vi "Actor Core.vi"(8 "error in":errorcluster, 11 "UI Actor in":refnum<class "UI Actor.lvclass">) -> (0 "error out":errorcluster, 3 "Actor out":refnum<class "Actor.lvclass">)   [LabVIEW 2024, in "UI Actor.lvlib" / "UI Actor.lvclass"]
doc: "<p>(<strong>Filename</strong>: <span class=\"dnl\">Actor Framework.lvlib:Actor.lvclass:Actor Core.vi</span>)</p>\n<p>Receives messages to the actor, reacts to them, and initiates any error handling that may shut the actor down.</p>\n<p>Descendant classes may override this VI to append parallel tasks for the actor to complete while it handles messages. Overrides use the <a href=\"nihelplauncher://docs/csh?context=lvcore_glang_udclass\">Call Parent Class Method</a> node.</p>"
uses:
  UI Actor.lvclass
  C:/Program Files/National Instruments/LabVIEW 2025/vi.lib/MGI/Panel Manager/Panel Actor/Panel Actor/Panel Actor.lvclass
  <vilib>/ActorFramework/Actor/Actor.lvclass
  Controls/Device Info.ctl
  Controls/File Info.ctl
  Controls/Device Settings.ctl
  Controls/Supported Baudrates.ctl
  Core/Object Type.ctl
  Core/Access SDO.ctl
  Core/Access PDO.ctl
  Core/Access SRDO.ctl
  D:/git/Sourcegrid-LabVIEW/dll/SourceGrid.dll
  Sourcegrid-LabVIEW/dll/SourceGrid.dll
  Controls/TX Communication Parameter.ctl
  Controls/RX Communication Parameter.ctl
  Sourcegrid-LabVIEW/source/MouseEventArgs/MouseEventArgs.lvclass
  <vilib>/MGI/Panel Manager/Panel/Panel Helper/Panel Events.ctl
  <vilib>/MGI/Panel Manager/Panel/Panel Helper/Events.ctl
  PDO Grid/PDO Grid.lvclass
  D:/git/Sourcegrid-LabVIEW/source/Grid/SourceGrid.lvclass
  <vilib>/Utility/miscctls.llb/LVRowAndColumnTypeDef.ctl
  UI Actor.lvclass/UI Actor.ctl
  Sourcegrid-LabVIEW/source/Grid/SourceGrid.lvclass/SourceGrid.ctl
  UI Actor Messages/Populate Attribute Details Msg/Populate Attribute Details Msg.lvclass/Populate Attribute Details Msg.ctl
  <vilib>/ActorFramework/Message Enqueuer/Message Enqueuer.lvclass/Message Enqueuer.ctl
  UI Actor Messages/Populate Attributes Table Msg/Populate Attributes Table Msg.lvclass/Populate Attributes Table Msg.ctl
  UI Actor Messages/Update TX Slot Display Msg/Update TX Slot Display Msg.lvclass/Update TX Slot Display Msg.ctl
  UI Actor Messages/Update RX Slot Display Msg/Update RX Slot Display Msg.lvclass/Update RX Slot Display Msg.ctl
  UI Actor Messages/Read EDS File Msg/Read EDS File Msg.lvclass/Read EDS File Msg.ctl
  <vilib>/ActorFramework/Message Enqueuer/Enqueue.vi
  UI Actor Messages/Populate Attribute Details Msg/Populate Attribute Details Msg.lvclass
  C:/Program Files/National Instruments/LabVIEW 2025/vi.lib/ActorFramework/Message/Message.lvclass
  UI Actor Messages/Populate Attributes Table Msg/Populate Attributes Table Msg.lvclass
  UI Actor Messages/Update TX Slot Display Msg/Update TX Slot Display Msg.lvclass
  UI Actor Messages/Update RX Slot Display Msg/Update RX Slot Display Msg.lvclass
  UI Actor Messages/Read EDS File Msg/Read EDS File Msg.lvclass
  <vilib>/ActorFramework/Stop Msg/Stop Msg.lvclass
  <vilib>/Utility/LVClass/Get LV Class Name.vi
  <vilib>/ActorFramework/tracing/Trace Generation/Generate Trace for Message.vi
  <vilib>/ActorFramework/Message Priority Queue/Priority Enqueue.vi
  Sourcegrid-LabVIEW/source/MouseEventArgs/Get Button.vi
  Sourcegrid-LabVIEW/source/MouseEventArgs/Get Location.vi
  <vilib>/MGI/Panel Manager/Panel Actor/Panel Actor/Panel Actor.lvclass
  UI Actor.lvlib
  Core/Electronic Datasheet.lvlib
  Sourcegrid-LabVIEW/source/Grid/SourceGrid.lvclass
  <vilib>/MGI/Panel Manager/Panel/Panel Helper/Panel Helper.lvclass
panel:
  in  "Filenames":i32(listbox)
  in  "Tab Control":T1(tab)
  out "auto":bool
  in  "Update Button":bool
  out "Concrete Node ID":string
  out "Device Settings":T2
  out "PDOs":T3
  out "File Info":T4
  out "DeviceInfo":T5
  out "Baudrates":T6
  in  "DefaultValue":string
  in  "Actual Value":string
  in  "Access SRDO":T7
  in  "Access PDO":T8
  in  "Access SDO":T9
  in  "LowLimit":string
  in  "HighLimit":string
  in  "DataType":u16(ring) items=["BOOLEAN"=1, "INTEGER8"=2, "INTEGER16"=3, "INTEGER32"=4, "UNSIGNED8"=5, "UNSIGNED16"=6, "UNSIGNED32"=7, "REAL32"=8, "VISIBLE_STRING"=9, "OCTET_STRING"=10, "UNICODE_STRING"=11, "TIME_OF_DAY"=12, "TIME_DIFFERENCE"=13, "RESERVED1"=14, "DOMAIN"=15, "INTEGER24"=16, "REAL64"=17, "INTEGER40"=18, "INTEGER48"=19, "INTEGER56"=20, "INTEGER64"=21, "UNSIGNED24"=22, "RESERVED2"=23, "UNSIGNED40"=24, "UNSIGNED48"=25, "UNSIGNED56"=26, "UNSIGNED64"=27, "RESERVED3"=28, "RESERVED4"=29, "RESERVED5"=30, "RESERVED6"=31, "PDO_COMMUNICATION_PARAMETER"=32, "PDO_MAPPING"=33, "SDO_PARAMETER"=34, "IDENTITY"=35, "RESERVED7"=36]
  out "ObjectType":T10 items=["NULL"=0, "DOMAIN"=2, "DEFTYPE"=5, "DEFSTRUCT"=6, "VAR"=7, "ARRAY"=8, "RECORD"=9]
  out "Sub-Index":string
  out "Index":string
  out "Attribute Table":string[][](table)
  out "Device Profile Specific":string[][](table)
  out "Manufacturer Specific":string[][](table)
  out "Communication Specific":string[][](table)
  in  "ParameterName":string
  in  "Description":string
  in  "Denotation":string
  in  "TX PDO Grid":refnum<k24>(container)
  out "Available Objects for TX PDO":string[][](table)
  out "TX Communication Parameter":T11 {"Type" items=["synchronous (acyclic)"=0, "synchronous (cyclic every sync)"=1, "synchronous (cyclic every 2nd SYNC)"=2, "synchronous (cyclic every 3rd SYNC)"=3, "synchronous (cyclic every 4th SYNC)"=4, "synchronous (cyclic every 240th SYNC)"=240, "reserved"=241, "reserved"=251, "RTR-only (synchronous)"=252, "RTR-only (event-driven)"=253, "event-driven (manufacturer-specific)"=254, "event-driven (device profile and application profile specific)"=255]; "COB" format="%.0x"; "Mapping" format="%.0x"; "Communication" format="%.0x"}
  in  "RX PDO Grid":refnum<k24>(container)
  out "RX Communication Parameters":T12={"Communication"=0, "Mapping"=0, "COB"=0, "Transm. Type"=254, "Inhibit"=0, "Event Timer"=0, "Sync Start"=0} {"Transm. Type" items=["synchronous"=0, "synchronous"=240, "reserved"=241, "reserved"=253, "event-driven (manufacturer-specific)"=254, "event-driven (device profile and application profile specific)"=255]; "COB" format="%.0x"; "Mapping" format="%.0x"; "Communication" format="%.0x"}
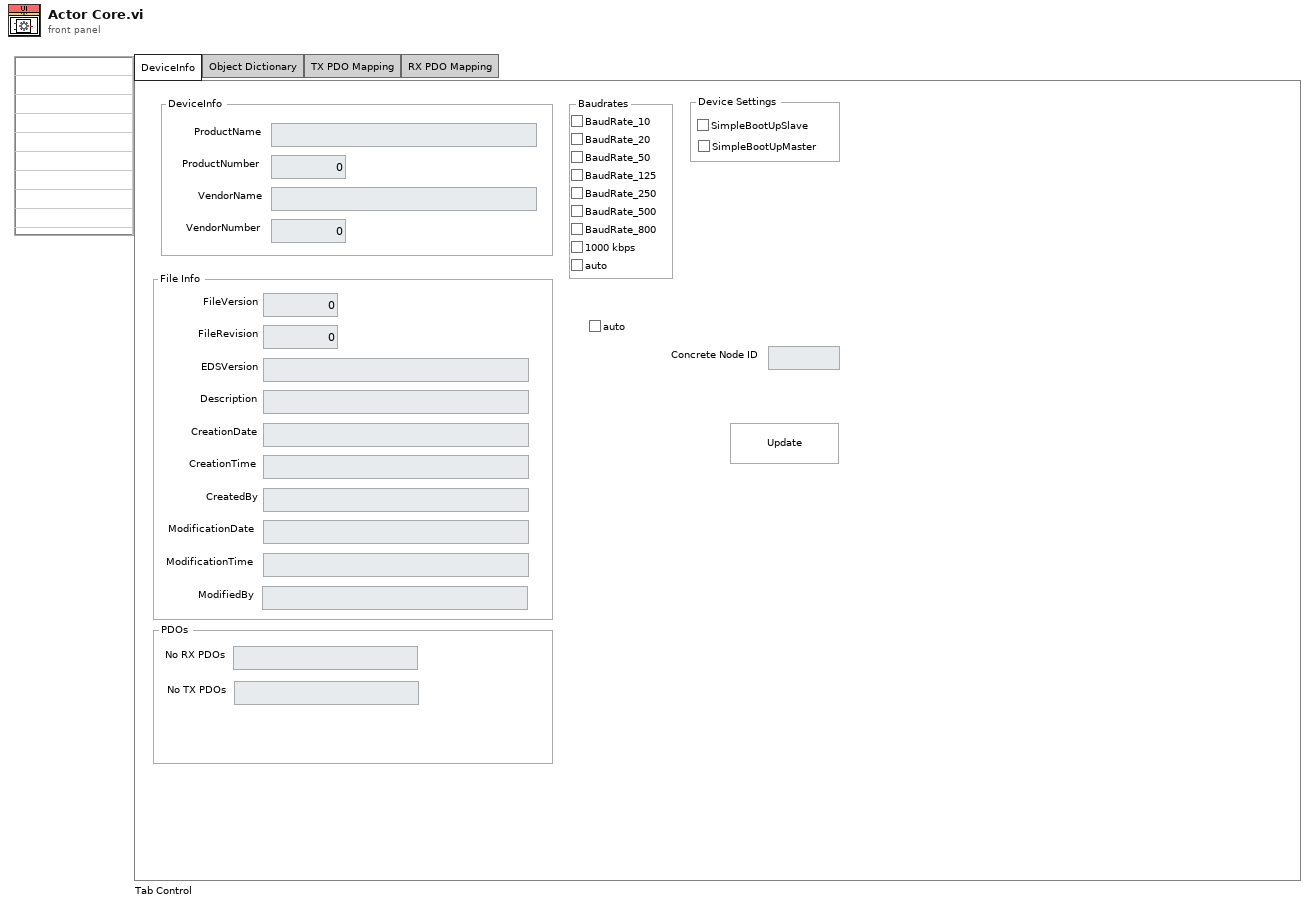
[diagram p1: front panel]
types:
  T1 = enum32{"DeviceInfo", "Object Dictionary", "TX PDO Mapping", "RX PDO Mapping"}
  T2 = typedef "UI Actor.lvlib/Device Settings.ctl" = cluster{"SimpleBootUpSlave":bool, "SimpleBootUpMaster":bool}
  T3 = cluster{"No RX PDOs":string, "No TX PDOs":string}
  T4 = typedef "UI Actor.lvlib/File Info.ctl" = cluster{"FileVersion":u8, "FileRevision":u8, "EDSVersion":string, "Description":string, "CreationDate":string, "CreationTime":string, "CreatedBy":string, "ModificationDate":string, "ModificationTime":string, "ModifiedBy":string}
  T5 = typedef "UI Actor.lvlib/Device Info.ctl" = cluster{"ProductName":string, "ProductNumber":u32, "VendorName":string, "VendorNumber":u32}
  T6 = typedef "UI Actor.lvlib/Supported Baudrates.ctl" = cluster{"BaudRate_10":bool, "BaudRate_20":bool, "BaudRate_50":bool, "BaudRate_125":bool, "BaudRate_250":bool, "BaudRate_500":bool, "BaudRate_800":bool, "BaudRate_1000":bool, "BaudRate_auto":bool}
  T7 = typedef "Electronic Datasheet.lvlib/Access SRDO.ctl" = enum16{"no", "tx", "rx", "trx"}
  T8 = typedef "Electronic Datasheet.lvlib/Access PDO.ctl" = enum16{"no", "TPDO", "RPDO", "TPDO & RPDO"}
  T9 = typedef "Electronic Datasheet.lvlib/Access SDO.ctl" = enum16{"read only", "write only", "read/write", "read/write on process input", "read/write on process output", "constant value", "no", "UNKNOWN"}
  T10 = typedef "Electronic Datasheet.lvlib/Object Type.ctl" = u8
  T11 = typedef "UI Actor.lvlib/UI Actor.lvclass/TX Communication Parameter.ctl" = cluster{"Communication":u16, "Mapping":u16, "COB":u32, "Type":u8, "Inhibit":u16, "Event Timer":u16, "Sync Start":u8}
  T12 = typedef "UI Actor.lvlib/UI Actor.lvclass/RX Communication Parameter.ctl" = cluster{"Communication":u16, "Mapping":u16, "COB":u32, "Transm. Type":u8, "Inhibit":u16, "Event Timer":u16, "Sync Start":u8}
  T13 = cluster{"Pnl Actor":refnum<event-registration>, "UI":refnum<event-registration>}
  T14 = typedef "LVRowAndColumnTypeDef.ctl" = cluster{"Row":i32, "Column":i32}
  T15 = cluster{"DeviceInfo":refnum<user-event>, "Baudrates":refnum<user-event>, "File Info":refnum<user-event>, "Device Settings":refnum<user-event>, "Filenames":refnum<user-event>, "Communication Specific":refnum<user-event>, "Manufacturer Specific":refnum<user-event>, "Device Profile Specific":refnum<user-event>, "Attribute Table":refnum<user-event>, "Attribute Details":refnum<user-event>, "TX Communication Parameter":refnum<user-event>, "RX Communication Parameter":refnum<user-event>, "Available Objects for TPDO":refnum<user-event>, "Available Objects for RPDO":refnum<user-event>}
  T16 = enum8{"Enabled", "Disabled", "Disabled and Grayed Out"}
  T17 = typedef "Rendezvous RefNum" = refnum<k1>
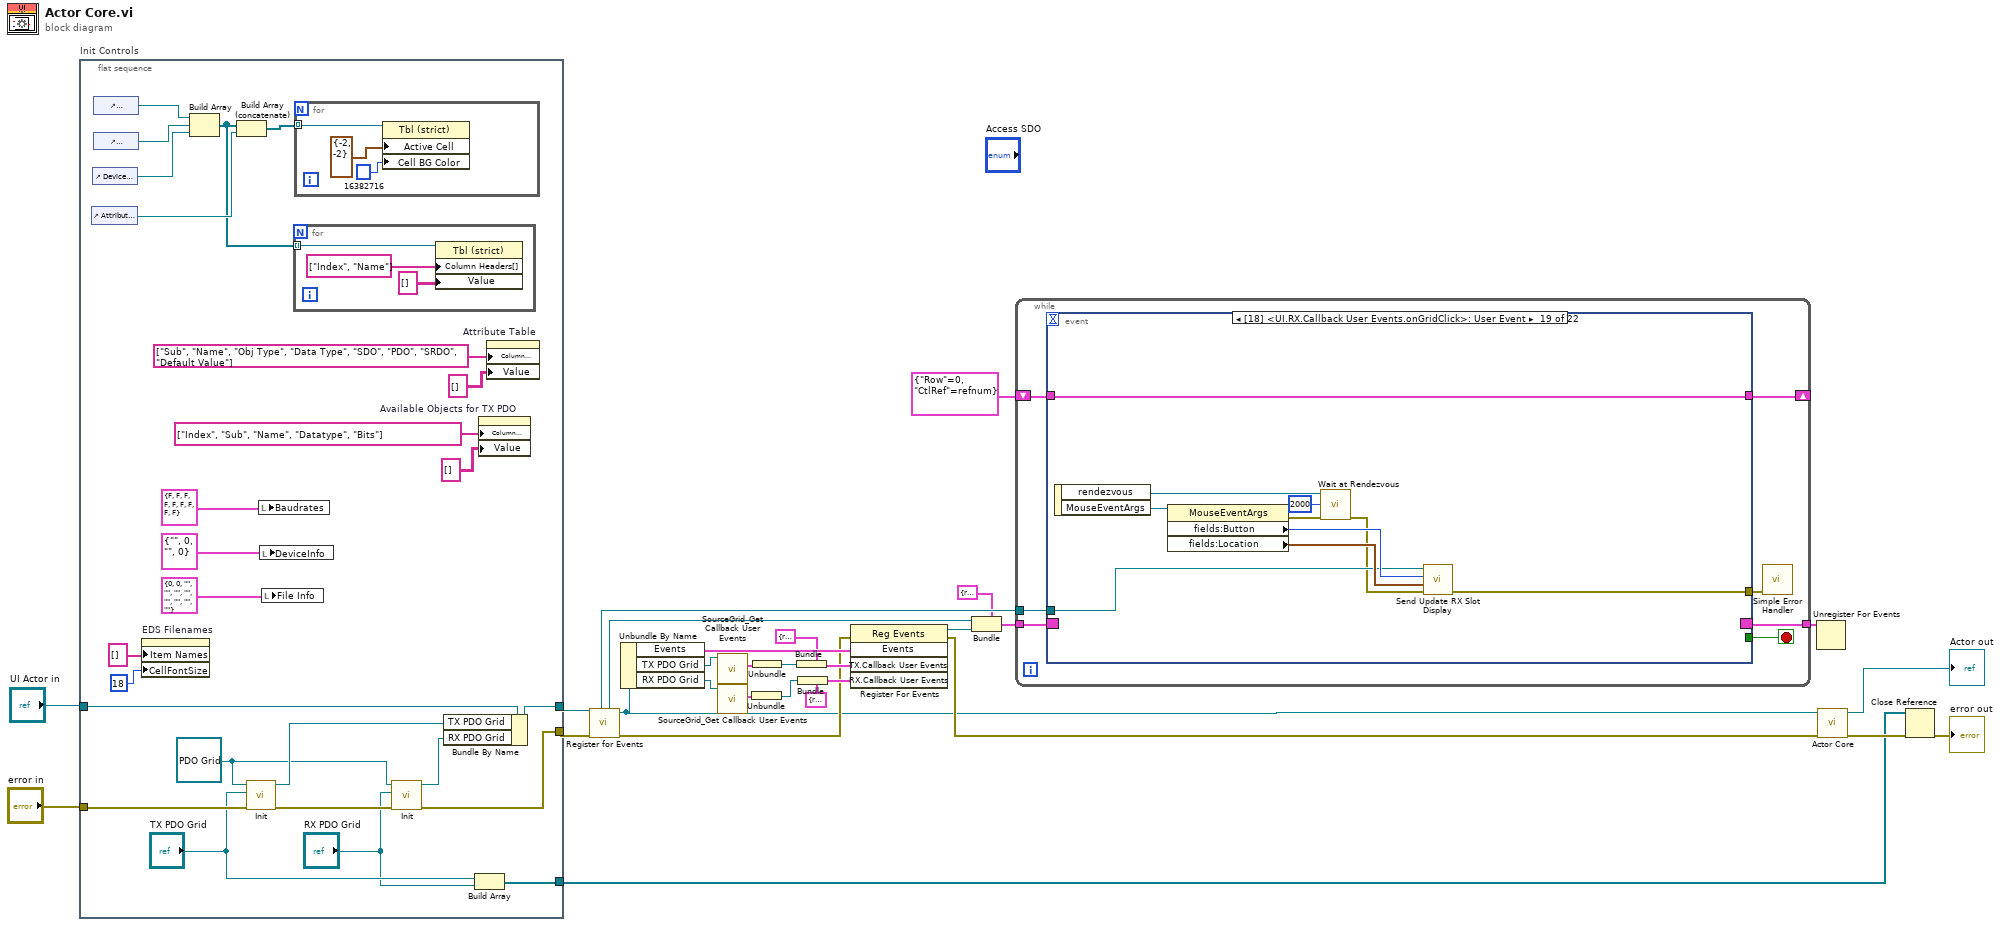
[diagram p0: block diagram]
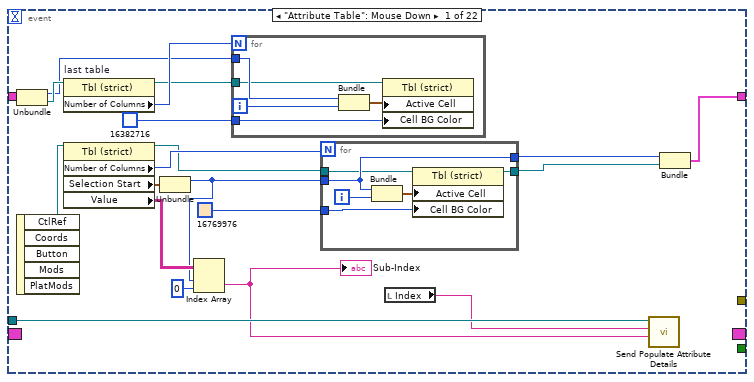
[diagram p2: hidden frame]
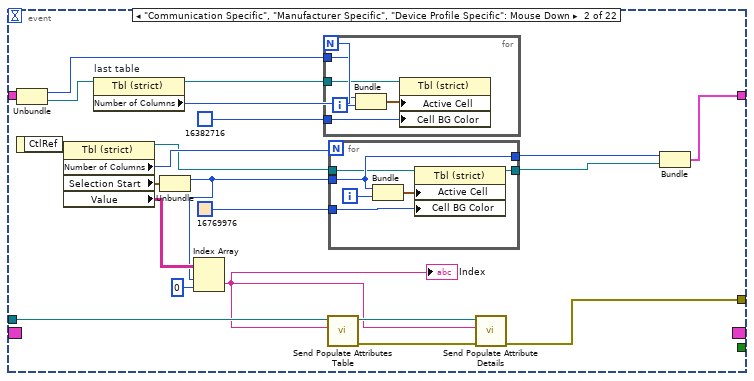
[diagram p3: hidden frame]
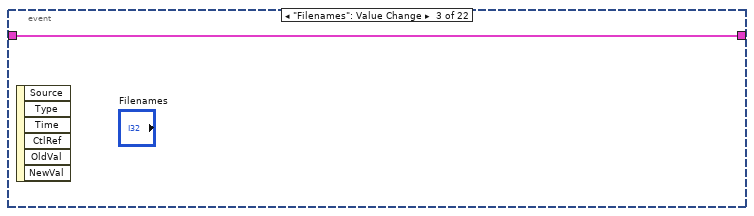
[diagram p4: hidden frame]
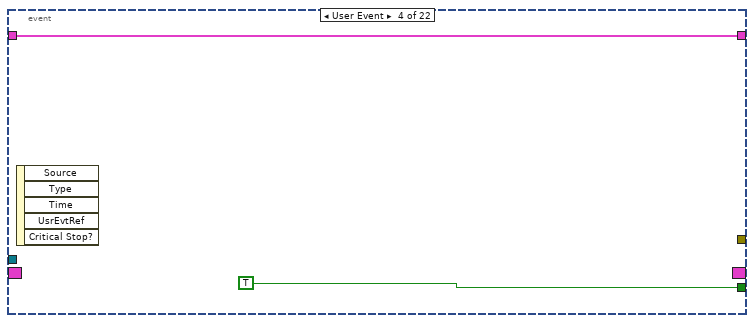
[diagram p5: hidden frame]
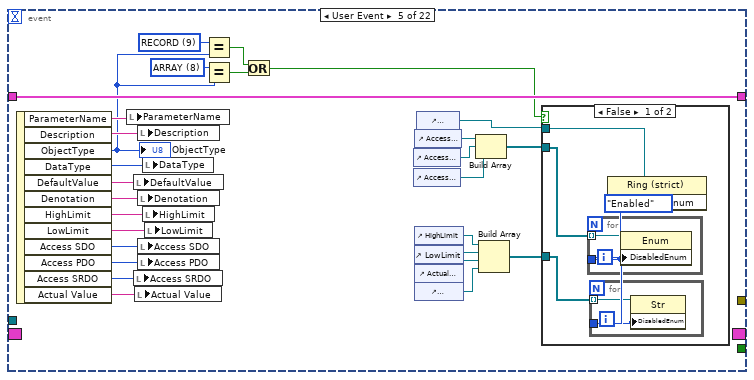
[diagram p6: hidden frame]
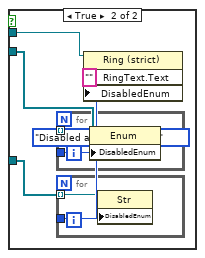
[diagram p7: hidden frame]
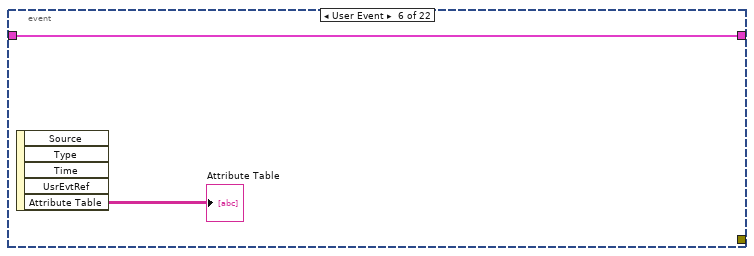
[diagram p8: hidden frame]
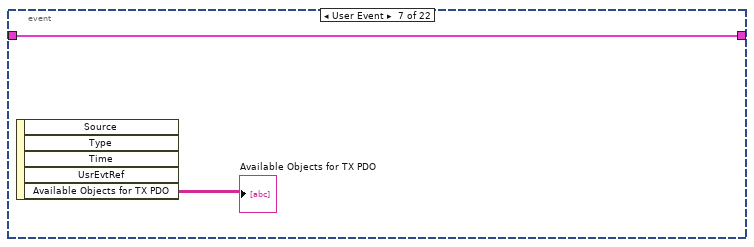
[diagram p9: hidden frame]
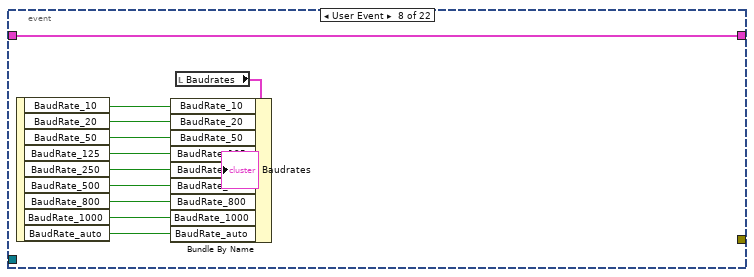
[diagram p10: hidden frame]
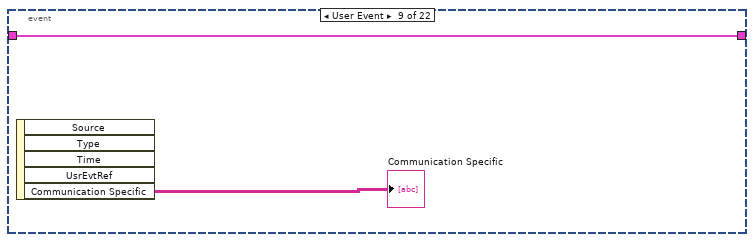
[diagram p11: hidden frame]
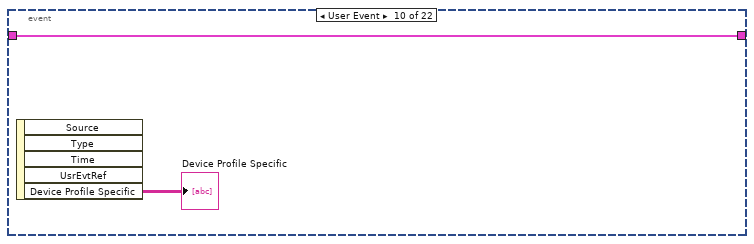
[diagram p12: hidden frame]
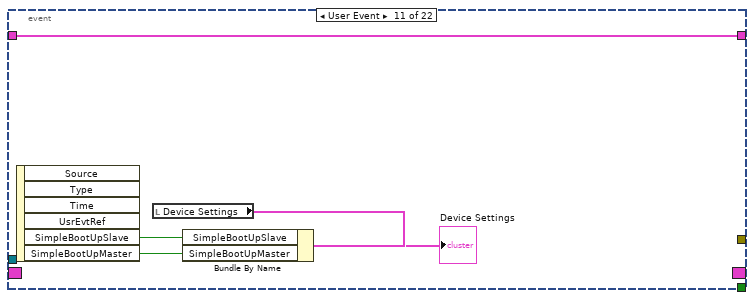
[diagram p13: hidden frame]
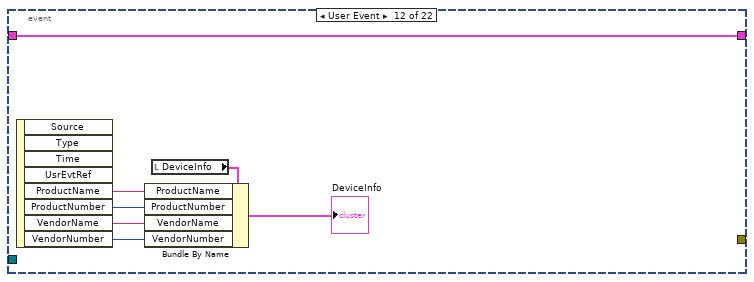
[diagram p14: hidden frame]
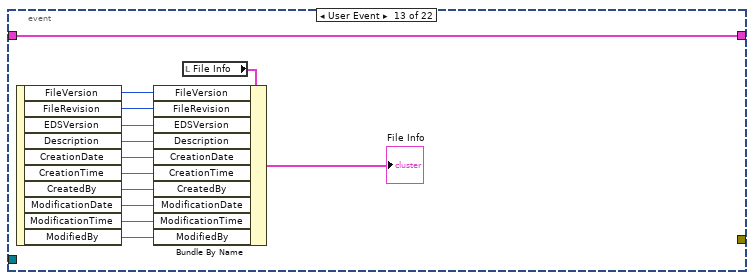
[diagram p15: hidden frame]
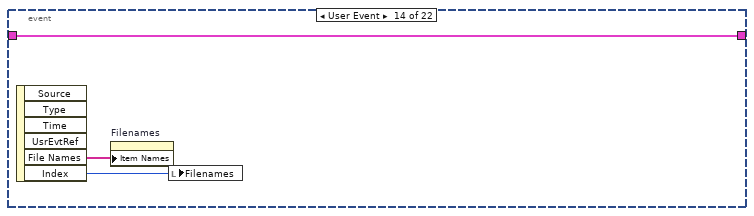
[diagram p16: hidden frame]
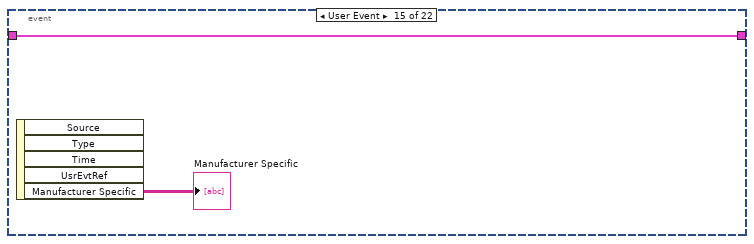
[diagram p17: hidden frame]
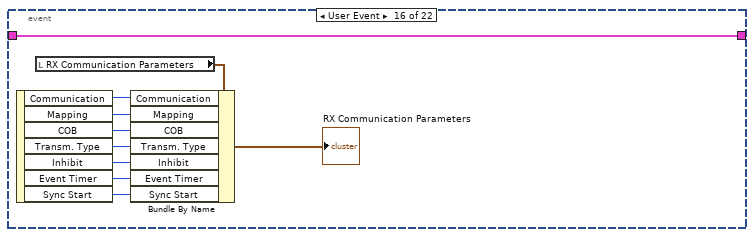
[diagram p18: hidden frame]
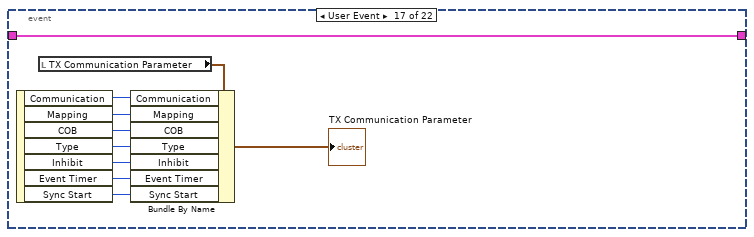
[diagram p19: hidden frame]
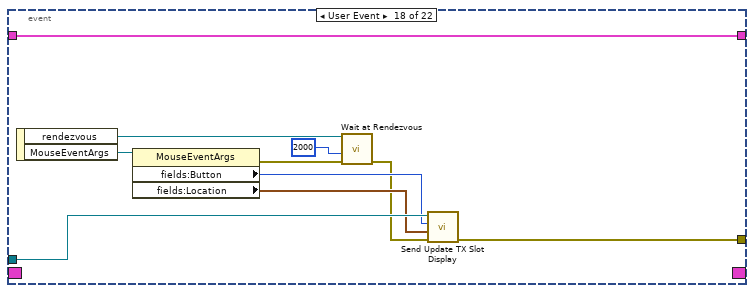
[diagram p20: hidden frame]
diagram:
  n1 = flat-sequence "Init Controls" {
    tunnel: "error in" -> [w42]
    tunnel: "UI Actor in" -> [w41]
    tunnel: [w37] -> w21
    tunnel: [w40] -> w20
    tunnel: [w30] -> w1
    frame #0 {
      w36 = refnum<class "PDO Grid.lvclass"> refnum ("PDO Grid.lvlib:PDO Grid.lvclass")
      n2 = control-ref of="Attribute Table"() -> (w44:refnum<vi>)
      n3 = control-ref of="Device Profile Specific"() -> (w46:refnum<vi>)
      n4 = control-ref of="Communication Specific"() -> (w48:refnum<vi>)
      n5 = control-ref of="Manufacturer Specific"() -> (w47:refnum<vi>)
      n6 = property on="EDS Filenames" class="LstBox (strict)"("Item Names"=string[] [], "CellFontSize"=u32 18 ("Size:Height")) -> ()  [unwired: 2 in, 2 out]
      n7 = Build Array(w48, w47, w46) -> (w43:refnum<vi>[])
      n8 = Build Array (concatenate)(w43, w44) -> (w45:refnum<vi>[])
      n9 = call-dynamic "Init.vi"("error in"=w42, "Sourcegrid Container"="TX PDO Grid", "PDO Grid in"=w36) -> ("error out"=w39:errorcluster, "PDO Grid out"=w38:refnum<class "PDO Grid.lvclass">)  [unwired: 7 in]
      n10 = local write "Baudrates"(T6 {"BaudRate_10"=FALSE, "BaudRate_20"=FALSE, "BaudRate_50"=FALSE, "BaudRate_125"=FALSE, "BaudRate_250"=FALSE, "BaudRate_500"=FALSE, "BaudRate_800"=FALSE, "BaudRate_1000"=FALSE, "BaudRate_auto"=FALSE} ("Baudrates")) -> ()
      n11 = local write "DeviceInfo"(T5 {"ProductName"="", "ProductNumber"=0, "VendorName"="", "VendorNumber"=0} ("DeviceInfo")) -> ()
      n12 = local write "File Info"(T4 {"FileVersion"=0, "FileRevision"=0, "EDSVersion"="", "Description"="", "CreationDate"="", "CreationTime"="", "CreatedBy"="", "ModificationDate"="", "ModificationTime"="", "ModifiedBy"=""} ("File Info")) -> ()
      n13 = for {
        tunnel: w43 -> [w56] mode=indexing
        n14 = property on="Property Node" class="Tbl (strict)"(reference=w56, "Column Headers[]"=string[] ["Index", "Name"] ("Compulsory Objects"), "Value"=string[][] [] ("Communication Specific")) -> ()  [unwired: 1 in, 2 out]
      }
      n15 = for {
        tunnel: w45 -> [w61] mode=indexing
        n16 = property class="Tbl (strict)"(reference=w61, "Active Cell"=T14 {"Row"=-2, "Column"=-2} ("Active Cell:Active Cell"), "Cell BG Color"=u32 16382716 ("Active Cell:Cell Background Color")) -> ()  [unwired: 1 in, 2 out]
      }
      n17 = call-dynamic "Init.vi"("error in"=w39, "Sourcegrid Container"="RX PDO Grid", "PDO Grid in"=w36) -> ("error out"=w37:errorcluster, "PDO Grid out"=w35:refnum<class "PDO Grid.lvclass">)  [unwired: 7 in]
      n18 = Bundle By Name(cluster=w41, "TX PDO Grid"=w38, "RX PDO Grid"=w35) -> (w40:refnum<class "UI Actor.lvclass">)
      n19 = Build Array("TX PDO Grid", "RX PDO Grid") -> (w30:refnum<k24>[])
      n20 = property on="Available Objects for TX PDO" class="Tbl (strict)"("Column Headers[]"=string[] ["Index", "Sub", "Name", "Datatype", "Bits"] ("Column Header Strings[]"), "Value"=string[][] [] ("Available Objects for TX PDO")) -> ()  [unwired: 2 in, 2 out]
      n21 = property on="Attribute Table" class="Tbl (strict)"("Column Headers[]"=string[] ["Sub", "Name", "Obj Type", "Data Type", "SDO", "PDO", "SRDO", "Default Value"] ("Compulsory Objects"), "Value"=string[][] [] ("Communication Specific")) -> ()  [unwired: 2 in, 2 out]
    }
  }
  n22 = call <vilib>:"Register for Events.vi"("Error In"=w21, "Panel Actor in"=w20) -> ("Error Out"=w5:errorcluster, "Panel Actor out"=w3:refnum<class "UI Actor.lvclass">, "Pnl Actor"=w27:refnum<event-registration>, "Self Enqueuer"=w26:refnum<class "Message Enqueuer.lvclass">)  [unwired: 6 in]
  n23 = Unbundle By Name(w3) -> ("Events"=w24:T15, "TX PDO Grid"=w17:refnum<class "PDO Grid.lvclass">, "RX PDO Grid"=w16:refnum<class "PDO Grid.lvclass">)
  n24 = call "SourceGrid_Get Callback User Events.vi"("SourceGrid in"=w17) -> ("Callback User Events"=w10:cluster{"onGridClick":refnum<user-event>})  [unwired: 9 in, 1 out]
  n25 = call "SourceGrid_Get Callback User Events.vi"("SourceGrid in"=w16) -> ("Callback User Events"=w15:cluster{"onGridClick":refnum<user-event>})  [unwired: 9 in, 1 out]
  n26 = Unbundle(w15) -> ("onGridClick"=w13:refnum<user-event>)
  n27 = Unbundle(w10) -> ("onGridClick"=w9:refnum<user-event>)
  n28 = Bundle(cluster=cluster{"onGridClick":refnum<user-event>} {"onGridClick"=refnum} ("TX.Callback User Events"), "onGridClick"=w9) -> (w11:cluster{"onGridClick":refnum<user-event>})
  n29 = Bundle(cluster=cluster{"onGridClick":refnum<user-event>} {"onGridClick"=refnum} ("RX.Callback User Events"), "onGridClick"=w13) -> (w14:cluster{"onGridClick":refnum<user-event>})
  n30 = register-events(error in=w5, w24, w11, w14) -> (reference out=w7:refnum<event-registration>, error out=w4:errorcluster)  [unwired: 1 in]
  n31 = Bundle(cluster=T13 {"Pnl Actor"=refnum, "UI"=refnum}, "Pnl Actor"=w27, "UI"=w7) -> (w25:T13)
  n32 = while {
    tunnel: w25 -> [w67]
    tunnel: w26 -> [w66]
    shift-right: [w65] -> _
    shift-left: cluster{"Row":i32, "CtlRef":refnum<vi>} {"Row"=0, "CtlRef"=refnum} -> [w64]
    tunnel: [w63] -> w18
    stop <- w68 stop-if-true
    n33 = event shown="[18] <UI.RX.Callback User Events.onGridClick>: User Event" {
      selector: w67 -> [_ _ _ _ _ _ _ _ _ _ _ _ _ _ _ _ _ _ _ _ _ _]
      dyn-events: [_ _ _ _ _ _ _ _ _ _ _ _ _ _ _ _ _ _ _ _ _ _] -> w63
      timeout: _ -> [_ _ _ _ _ _ _ _ _ _ _ _ _ _ _ _ _ _ _ _ _ _]
      tunnel: [_ _ _ TRUE _ _ _ _ _ _ _ _ _ _ _ _ _ _ _ _ _ _] -> w68
      tunnel: w66 -> [w73 w106 _ _ _ _ _ _ _ _ _ _ _ _ _ _ _ w258 w266 w273 w298 _]
      tunnel: [w78 w111 w133 w134 w163 w181 w183 w185 w198 w199 w201 w206 w213 w226 w229 w232 w241 w260 w264 w272 w297 w300] -> w65
      tunnel: w64 -> [w87 w120 w133 w134 w163 w181 w183 w185 w198 w199 w201 w206 w213 w226 w229 w232 w241 w260 w264 w272 w297 w300]
      tunnel: [_ w100 _ _ _ _ _ _ _ _ _ _ _ _ _ _ _ w256 w265 w271 _ _] -> w62
      event "Attribute Table": Mouse Down {
        n34 = Unbundle(w87) -> ("Row"=w79:i32, "CtlRef"=w80:refnum<vi>)
        n35 = event-data() -> ("CtlRef"=w75:refnum<vi>)  [unwired: 1 in, 4 out]
        n36 = property on="last table" class="Tbl (strict)"(reference=w80) -> (reference out=w76:refnum<vi>, "Number of Columns"=w81:u32)  [unwired: 1 in, 1 out]
        n37 = property class="Tbl (strict)"(reference=w75) -> (reference out=w83:refnum<vi>, "Number of Columns"=w86:u32, "Selection Start"=w88:T14, "Value"=w74:string[][])  [unwired: 1 in, 1 out]
        n38 = Unbundle(w88) -> ("Row"=w71:i32)  [unwired: 1 out]
        n39 = Index Array(array=w74, index (row)=w71, index (col)=0) -> (element=w69:string)
        "Sub-Index" <- w69
        n40 = for {
          N: w81 -> [_]
          tunnel: u32 16382716 ("Active Cell:Cell Background Color") -> [w99]
          tunnel: w79 -> [w96]
          tunnel: w76 -> [w95]
          i -> [w98]
          n41 = Bundle("Row"=w96, w98) -> (w97:cluster{"Row":i32, i32})  [unwired: 1 in]
          n42 = property class="Tbl (strict)"(reference=w95, "Active Cell"=w97, "Cell BG Color"=w99) -> ()  [unwired: 1 in, 2 out]
        }
        n43 = for {
          N: w86 -> [_]
          tunnel: w71 -> [w93]
          tunnel: u32 16769976 -> [w92]
          tunnel: [w93] -> w84
          tunnel: w83 -> [w90]
          tunnel: [w89] -> w77
          i -> [w94]
          n44 = Bundle("Row"=w93, w94) -> (w91:cluster{"Row":i32, i32})  [unwired: 1 in]
          n45 = property class="Tbl (strict)"(reference=w90, "Active Cell"=w91, "Cell BG Color"=w92) -> (reference out=w89:refnum<vi>)  [unwired: 1 in, 1 out]
        }
        n46 = local read "Index"() -> (w70:string)
        n47 = call "Send Populate Attribute Details.vi"("Sub-Index"=w69, "Index"=w70, "Message Enqueuer"=w73) -> ()  [unwired: 7 in, 2 out]
        n48 = Bundle("Row"=w84, "CtlRef"=w77) -> (w78:cluster{"Row":i32, "CtlRef":refnum<vi>})  [unwired: 1 in]
      }
      event "Communication Specific", "Manufacturer Specific", "Device Profile Specific": Mouse Down {
        n49 = Unbundle(w120) -> ("Row"=w112:i32, "CtlRef"=w113:refnum<vi>)
        n50 = event-data() -> ("CtlRef"=w108:refnum<vi>)  [unwired: 1 in]
        n51 = property class="Tbl (strict)"(reference=w108) -> (reference out=w116:refnum<vi>, "Number of Columns"=w119:u32, "Selection Start"=w121:T14, "Value"=w107:string[][])  [unwired: 1 in, 1 out]
        n52 = property on="last table" class="Tbl (strict)"(reference=w113) -> (reference out=w109:refnum<vi>, "Number of Columns"=w114:u32)  [unwired: 1 in, 1 out]
        n53 = Unbundle(w121) -> ("Row"=w104:i32)  [unwired: 1 out]
        n54 = Index Array(array=w107, index (row)=w104, index (col)=0) -> (element=w102:string)
        "Index" <- w102
        n55 = for {
          N: w114 -> [_]
          tunnel: u32 16382716 ("Active Cell:Cell Background Color") -> [w132]
          tunnel: w112 -> [w129]
          tunnel: w109 -> [w128]
          i -> [w131]
          n56 = Bundle("Row"=w129, w131) -> (w130:cluster{"Row":i32, i32})  [unwired: 1 in]
          n57 = property class="Tbl (strict)"(reference=w128, "Active Cell"=w130, "Cell BG Color"=w132) -> ()  [unwired: 1 in, 2 out]
        }
        n58 = call "Send Populate Attributes Table.vi"("Index"=w102, "Message Enqueuer"=w106) -> ("error out"=w101:errorcluster, "Message Enqueuer out"=w103:refnum<class "Message Enqueuer.lvclass">)  [unwired: 8 in]
        n59 = for {
          N: w119 -> [_]
          tunnel: w104 -> [w126]
          tunnel: u32 16769976 -> [w125]
          tunnel: [w126] -> w117
          tunnel: w116 -> [w123]
          tunnel: [w122] -> w110
          i -> [w127]
          n60 = Bundle("Row"=w126, w127) -> (w124:cluster{"Row":i32, i32})  [unwired: 1 in]
          n61 = property class="Tbl (strict)"(reference=w123, "Active Cell"=w124, "Cell BG Color"=w125) -> (reference out=w122:refnum<vi>)  [unwired: 1 in, 1 out]
        }
        n62 = call "Send Populate Attribute Details.vi"("error in (no error)"=w101, "Index"=w102, "Message Enqueuer"=w103) -> ("error out"=w100:errorcluster)  [unwired: 7 in, 1 out]
        n63 = Bundle("Row"=w117, "CtlRef"=w110) -> (w111:cluster{"Row":i32, "CtlRef":refnum<vi>})  [unwired: 1 in]
      }
      event "Filenames": Value Change {
        n64 = event-data() -> ()  [unwired: 1 in, 6 out]
      }
      event User Event {
        n65 = event-data() -> ()  [unwired: 1 in, 5 out]
      }
      event User Event {
        w147 = T10 9 items=["NULL"=0, "DOMAIN"=2, "DEFTYPE"=5, "DEFSTRUCT"=6, "VAR"=7, "ARRAY"=8, "RECORD"=9] ("x")
        w148 = T10 8 items=["NULL"=0, "DOMAIN"=2, "DEFTYPE"=5, "DEFSTRUCT"=6, "VAR"=7, "ARRAY"=8, "RECORD"=9] ("x")
        n66 = event-data() -> ("ParameterName"=w162:string, "Description"=w161:string, "ObjectType"=w149:T10, "DataType"=w160:u16, "DefaultValue"=w159:string, "Denotation"=w158:string, "HighLimit"=w157:string, "LowLimit"=w156:string, "Access SDO"=w155:T9, "Access PDO"=w154:T8, "Access SRDO"=w153:T7, "Actual Value"=w152:string)  [unwired: 1 in]
        "ObjectType" <- w149
        n67 = local write "ParameterName"(w162) -> ()
        n68 = local write "DefaultValue"(w159) -> ()
        n69 = local write "Access SRDO"(w153) -> ()
        n70 = local write "Actual Value"(w152) -> ()
        n71 = local write "Description"(w161) -> ()
        n72 = local write "Denotation"(w158) -> ()
        n73 = local write "Access SDO"(w155) -> ()
        n74 = local write "Access PDO"(w154) -> ()
        n75 = local write "DataType"(w160) -> ()
        n76 = local write "HighLimit"(w157) -> ()
        n77 = local write "LowLimit"(w156) -> ()
        n78 = Equal?(x=w147, y=w149) -> (x = y?=w150:bool)
        n79 = Equal?(x=w148, y=w149) -> (x = y?=w151:bool)
        n80 = Or(x=w150, y=w151) -> (x .or. y?=w137:bool)
        n81 = control-ref of="Access PDO"() -> (w145:refnum<vi>)
        n82 = control-ref of="Access SRDO"() -> (w144:refnum<vi>)
        n83 = control-ref of="Access SDO"() -> (w146:refnum<vi>)
        n84 = control-ref of="HighLimit"() -> (w139:refnum<vi>)
        n85 = control-ref of="LowLimit"() -> (w140:refnum<vi>)
        n86 = control-ref of="Actual Value"() -> (w141:refnum<vi>)
        n87 = control-ref of="DefaultValue"() -> (w142:refnum<vi>)
        n88 = control-ref of="ObjectType"() -> (w136:refnum<vi>)
        n89 = Build Array(w146, w145, w144) -> (w143:refnum<vi>[])
        n90 = Build Array(w139, w140, w141, w142) -> (w138:refnum<vi>[])
        n91 = case shown="False" w137 {
          tunnel: w143 -> [w166 w176]
          tunnel: w138 -> [w167 w175]
          tunnel: w136 -> [w165 w174]
          frame False {
            w164 = T16."Enabled" ("Disabled")
            n92 = for {
              tunnel: w166 -> [w171] mode=indexing
              tunnel: w164 -> [w170]
              n93 = property on="Property Node" class="Enum"(reference=w171, "DisabledEnum"=w170) -> ()  [unwired: 1 in, 2 out]
            }
            n94 = for {
              tunnel: w167 -> [w169] mode=indexing
              tunnel: w164 -> [w168]
              n95 = property on="Property Node" class="Str"(reference=w169, "DisabledEnum"=w168) -> ()  [unwired: 1 in, 2 out]
            }
            n96 = property on="Property Node" class="Ring (strict)"(reference=w165, "DisabledEnum"=w164) -> ()  [unwired: 1 in, 2 out]
          }
          frame True {
            w172 = T16."Disabled and Grayed Out" ("Disabled")
            n97 = for {
              tunnel: w176 -> [w180] mode=indexing
              tunnel: w172 -> [w179]
              n98 = property on="Property Node" class="Enum"(reference=w180, "DisabledEnum"=w179) -> ()  [unwired: 1 in, 2 out]
            }
            n99 = for {
              tunnel: w175 -> [w178] mode=indexing
              tunnel: w172 -> [w177]
              n100 = property on="Property Node" class="Str"(reference=w178, "DisabledEnum"=w177) -> ()  [unwired: 1 in, 2 out]
            }
            n101 = property on="Property Node" class="Ring (strict)"(reference=w174, "RingText.Text"="" ("Ring Text.Text"), "DisabledEnum"=w172) -> ()  [unwired: 1 in, 2 out]
          }
        }
      }
      event User Event {
        n102 = event-data() -> ("Attribute Table"=→"Attribute Table":string[][])  [unwired: 1 in, 4 out]
      }
      event User Event {
        n103 = event-data() -> ("Available Objects for TX PDO"=→"Available Objects for TX PDO":string[][])  [unwired: 1 in, 4 out]
      }
      event User Event {
        n104 = event-data() -> ("BaudRate_10"=w195:bool, "BaudRate_20"=w194:bool, "BaudRate_50"=w193:bool, "BaudRate_125"=w192:bool, "BaudRate_250"=w191:bool, "BaudRate_500"=w190:bool, "BaudRate_800"=w189:bool, "BaudRate_1000"=w188:bool, "BaudRate_auto"=w186:bool)  [unwired: 1 in]
        n105 = local read "Baudrates"() -> (w196:T6)
        n106 = Bundle By Name(cluster=w196, "BaudRate_10"=w195, "BaudRate_20"=w194, "BaudRate_50"=w193, "BaudRate_125"=w192, "BaudRate_250"=w191, "BaudRate_500"=w190, "BaudRate_800"=w189, "BaudRate_1000"=w188, "BaudRate_auto"=w186) -> (→"Baudrates":T6)
      }
      event User Event {
        n107 = event-data() -> ("Communication Specific"=→"Communication Specific":string[][])  [unwired: 1 in, 4 out]
      }
      event User Event {
        n108 = event-data() -> ("Device Profile Specific"=→"Device Profile Specific":string[][])  [unwired: 1 in, 4 out]
      }
      event User Event {
        n109 = event-data() -> ("SimpleBootUpSlave"=w204:bool, "SimpleBootUpMaster"=w203:bool)  [unwired: 1 in, 4 out]
        n110 = local read "Device Settings"() -> (w205:T2)
        n111 = Bundle By Name(cluster=w205, "SimpleBootUpSlave"=w204, "SimpleBootUpMaster"=w203) -> (→"Device Settings":T2)
      }
      event User Event {
        n112 = event-data() -> ("ProductName"=w211:string, "ProductNumber"=w210:u32, "VendorName"=w209:string, "VendorNumber"=w208:u32)  [unwired: 1 in, 4 out]
        n113 = local read "DeviceInfo"() -> (w212:T5)
        n114 = Bundle By Name(cluster=w212, "ProductName"=w211, "ProductNumber"=w210, "VendorName"=w209, "VendorNumber"=w208) -> (→"DeviceInfo":T5)
      }
      event User Event {
        n115 = event-data() -> ("FileVersion"=w215:u8, "FileRevision"=w216:u8, "EDSVersion"=w217:string, "Description"=w218:string, "CreationDate"=w219:string, "CreationTime"=w220:string, "CreatedBy"=w221:string, "ModificationDate"=w222:string, "ModificationTime"=w223:string, "ModifiedBy"=w224:string)  [unwired: 1 in]
        n116 = local read "File Info"() -> (w225:T4)
        n117 = Bundle By Name(cluster=w225, "FileVersion"=w215, "FileRevision"=w216, "EDSVersion"=w217, "Description"=w218, "CreationDate"=w219, "CreationTime"=w220, "CreatedBy"=w221, "ModificationDate"=w222, "ModificationTime"=w223, "ModifiedBy"=w224) -> (→"File Info":T4)
      }
      event User Event {
        n118 = event-data() -> ("File Names"=w228:string[], "Index"=w227:i32)  [unwired: 1 in, 4 out]
        n119 = property on="Filenames" class="LstBox (strict)"("Item Names"=w228) -> ()  [unwired: 2 in, 2 out]
        n120 = local write "Filenames"(w227) -> ()
      }
      event User Event {
        n121 = event-data() -> ("Manufacturer Specific"=→"Manufacturer Specific":string[][])  [unwired: 1 in, 4 out]
      }
      event User Event {
        n122 = event-data() -> ("Communication"=w239:u16, "Mapping"=w238:u16, "COB"=w237:u32, "Transm. Type"=w236:u8, "Inhibit"=w235:u16, "Event Timer"=w234:u16, "Sync Start"=w233:u8)  [unwired: 1 in]
        n123 = local read "RX Communication Parameters"() -> (w240:T12)
        n124 = Bundle By Name(cluster=w240, "Communication"=w239, "Mapping"=w238, "COB"=w237, "Transm. Type"=w236, "Inhibit"=w235, "Event Timer"=w234, "Sync Start"=w233) -> (→"RX Communication Parameters":T12)
      }
      event User Event {
        n125 = event-data() -> ("Communication"=w249:u16, "Mapping"=w248:u16, "COB"=w247:u32, "Type"=w246:u8, "Inhibit"=w245:u16, "Event Timer"=w244:u16, "Sync Start"=w243:u8)  [unwired: 1 in]
        n126 = local read "TX Communication Parameter"() -> (w250:T11)
        n127 = Bundle By Name(cluster=w250, "Communication"=w249, "Mapping"=w248, "COB"=w247, "Type"=w246, "Inhibit"=w245, "Event Timer"=w244, "Sync Start"=w243) -> (→"TX Communication Parameter":T11)
      }
      event User Event {
        n128 = event-data() -> ("rendezvous"=w252:T17, "MouseEventArgs"=w259:refnum<class "MouseEventArgs.lvclass">)  [unwired: 1 in]
        n129 = property class="MouseEventArgs"(reference=w259) -> (error out=w257:errorcluster, "fields:Button"=w255:i32, "fields:Location"=w254:cluster{"X":i32, "Y":i32})  [unwired: 1 in, 1 out]
        n130 = call <vilib>:"Wait at Rendezvous.vi"("error in (no error)"=w257, "ms timeout (-1)"=2000, "rendezvous"=w252) -> ("error out"=w253:errorcluster)  [unwired: 2 in, 2 out]
        n131 = call "Send Update TX Slot Display.vi"("error in (no error)"=w253, "Location"=w254, "Button"=w255, "Message Enqueuer"=w258) -> ("error out"=w256:errorcluster)  [unwired: 6 in, 1 out]
      }
      event User Event {
        n132 = event-data() -> ("rendezvous"=w262:T17, "MouseEventArgs"=w267:refnum<class "MouseEventArgs.lvclass">)  [unwired: 1 in]
        n133 = property class="MouseEventArgs"(reference=w267) -> (error out=w270:errorcluster, "fields:Button"=w269:i32, "fields:Location"=w268:cluster{"X":i32, "Y":i32})  [unwired: 1 in, 1 out]
        n134 = call <vilib>:"Wait at Rendezvous.vi"("error in (no error)"=w270, "ms timeout (-1)"=2000, "rendezvous"=w262) -> ("error out"=w263:errorcluster)  [unwired: 2 in, 2 out]
        n135 = call "Send Update RX Slot Display.vi"("error in (no error)"=w263, "Location"=w268, "Button"=w269, "Message Enqueuer"=w266) -> ("error out"=w265:errorcluster)  [unwired: 6 in, 1 out]
      }
      event Menu Selection (User) {
        n136 = event-data() -> ("ItemPath"=w274:string)  [unwired: 1 in, 6 out]
        n137 = case shown="\"File:Open\"" w274 {
          tunnel: w273 -> [_ w286]
          tunnel: [_ w276] -> w271
          frame "False", Default {
          }
          frame "File:Open" {
            n138 = Current VI's Path() -> (path=w284:path)
            n139 = Strip Path(path=w284) -> (stripped path=w280:path)  [unwired: 1 out]
            n140 = Build Path(base path=w280, name or relative path=path "LastEdsPath.ini") -> (appended path=w278:path)
            n141 = Read from Text File(file (use dialog)=w278) -> (text=w283:string)  [unwired: 3 in, 3 out]
            n142 = String To Path(string=w283) -> (path=w282:path)
            n143 = call "File Dialog"("start path"=w282, "pattern (all files)"="*.eds") -> ("selected path"=w281:path, "cancelled"=w285:bool, "error out"=w288:errorcluster)  [unwired: 10 in, 1 out]
            n144 = case "Cancelled?" shown="False" w285 {
              tunnel: w288 -> [w291 w296]
              tunnel: w286 -> [w295 _]
              tunnel: w281 -> [w292 _]
              tunnel: w278 -> [w293 _]
              tunnel: [w289 w296] -> w277
              frame False {
                n145 = Path To String(path=w292) -> (string=w294:string)
                n146 = call "Send Read EDS File.vi"("error in (no error)"=w291, "EDS File Path"=w292, "Message Enqueuer"=w295) -> ("error out"=w290:errorcluster)  [unwired: 7 in, 1 out]
                n147 = Write to Text File(file (use dialog)=w293, text=w294, error in=w290) -> (error out=w289:errorcluster)  [unwired: 1 in, 2 out]
              }
              frame True {
              }
            }
            n148 = call <vilib>:"Clear Errors.vi"("error in (no error)"=w277, "specific error code to clear (0: all)"=43) -> ("error out"=w276:errorcluster)  [unwired: 4 in, 1 out]
          }
        }
      }
      event Panel Close? {
        n149 = event-data() -> ()  [unwired: 1 in, 4 out]
        n150 = call <vilib>:"Send Normal Stop.vi"("Message Enqueuer"=w298) -> ()  [unwired: 10 in, 1 out]
        n151 = event-data("Discard?"=TRUE) -> ()  [unwired: 1 in, 1 out]
      }
      event Timeout {
        n152 = event-data() -> ()  [unwired: 1 in, 3 out]
      }
    }
    n153 = call <vilib>:"Simple Error Handler.vi"("error in (no error)"=w62) -> ()  [unwired: 4 in, 5 out]
  }
  n154 = Unregister For Events(event registration refnum=w18) -> ()  [unwired: 1 in, 1 out]
  n155 = call-parent "Actor Core.vi"("error in"=w4, "Panel Actor in"=w3) -> ("error out"=w29:errorcluster, "Actor out"=→"Actor out":refnum<class "Actor.lvclass">)  [unwired: 8 in]
  n156 = Close Reference(reference=w1, error in (no error)=w29) -> (error out=→"error out":errorcluster)
